vi "Clear Entry.vi"(8 "error in (no error)":errorcluster, 10 "Key":string, 11 "FlexWorktable in":refnum<class "FlexWorktable.lvclass">) -> (0 "error out":errorcluster, 2 "Found":bool=TRUE, 3 "FlexWorktable out":refnum<class "FlexWorktable.lvclass">)   [LabVIEW 2017, in "FlexWorktable.lvclass"]
uses:
  FlexWorktable.lvclass
  FlexWorktable.lvclass/FlexWorktable.ctl
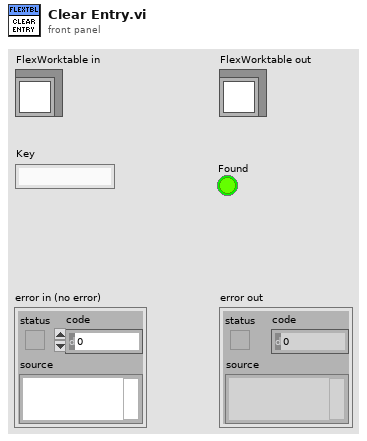
[diagram p1: front panel]
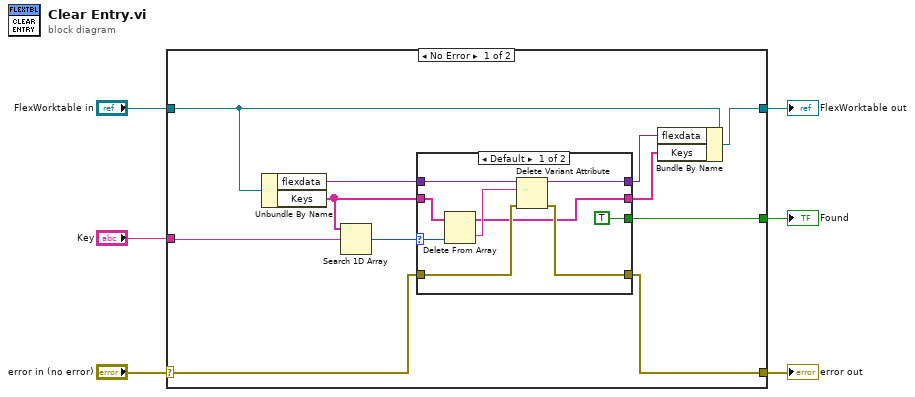
[diagram p0: block diagram]
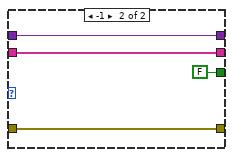
[diagram p2: hidden frame]
diagram:
  n1 = case shown="No Error" "error in (no error)" {
    selector: "error in (no error)" -> [w13 w32]
    tunnel: [w12 w32] -> w5
    tunnel: [w7 w31] -> w3
    tunnel: "FlexWorktable in" -> [w10 w31]
    tunnel: "Key" -> [w17 _]
    tunnel: [w11 _] -> w1
    frame No Error {
      n2 = Unbundle By Name(w10) -> ("flexdata"=w14:variant, "Keys"=w15:string[])
      n3 = Search 1D Array(1D array=w15, element=w17) -> (index of element=w16:i32)  [unwired: 1 in]
      n4 = case shown="Default" w16 {
        selector: w16 -> [w25 _]
        tunnel: w15 -> [w26 w27]
        tunnel: w14 -> [w24 w28]
        tunnel: [w22 w28] -> w9
        tunnel: w13 -> [w21 w30]
        tunnel: [w19 w30] -> w12
        tunnel: [TRUE FALSE] -> w11
        tunnel: [w18 w27] -> w8
        frame Default {
          n5 = Delete From Array(array=w26, index=w25) -> (deleted portion=w23:string, array with subset deleted=w18:string[])  [unwired: 1 in]
          n6 = Delete Variant Attribute(4:w21, 6:w23, 7:w24) -> (0:w19:errorcluster, 3:w22:variant)  [unwired: 1 out]
        }
        frame -1 {
        }
      }
      n7 = Bundle By Name(cluster=w10, "flexdata"=w9, "Keys"=w8) -> (w7:refnum<class "FlexWorktable.lvclass">)
    }
    frame Error {
    }
  }
  "error out" <- w5
  "FlexWorktable out" <- w3
  "Found" <- w1
